vi "Write Top Down Working Set.vi"(8 "error in (no error)":errorcluster, 10 "Top Down Working Set":refnum<data-value>, 11 "Build Analyzer in":refnum<class "Build Analyzer.lvclass">) -> (0 "error out":errorcluster, 3 "Build Analyzer out":refnum<class "Build Analyzer.lvclass">)   [LabVIEW 2017, in "CL_G3_VIComponentBuilder.lvlib" / "Build Analyzer.lvclass"]
doc: "Sets the hierarchy of components in the working set as a LabVIEW Container. Given a node in the tree, the children of this node are returned as dependents."
uses:
  Build Analyzer.lvclass
  <userlib>/_Cirrus Logic/LabVIEW Container/Source/Container/Container.lvclass
  Build Analyzer.lvclass/Build Analyzer.ctl
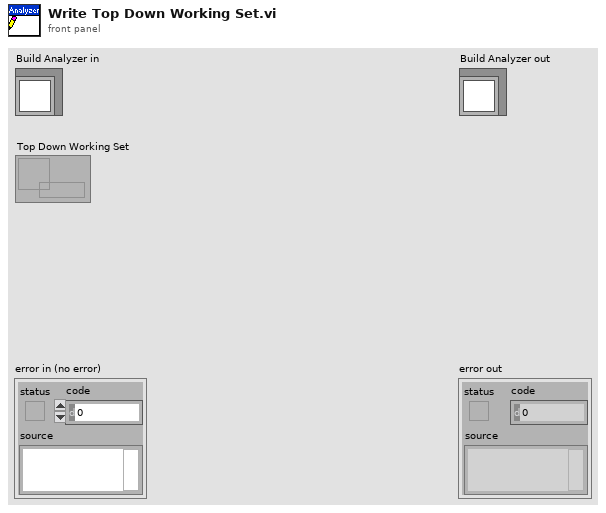
[diagram p1: front panel]
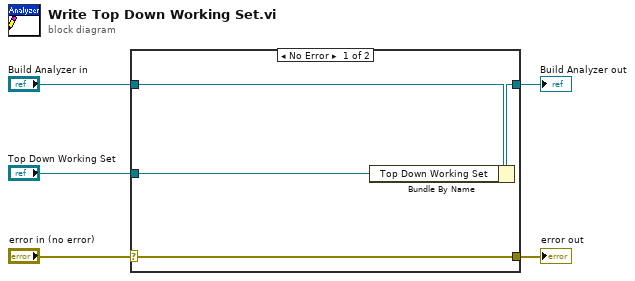
[diagram p0: block diagram]
diagram:
  n1 = case shown="No Error" "error in (no error)" {
    selector: "error in (no error)" -> [w9 w10]
    tunnel: [w9 w10] -> w4
    tunnel: [w7 w11] -> w2
    tunnel: "Build Analyzer in" -> [w8 w11]
    tunnel: "Top Down Working Set" -> [w6 _]
    frame No Error {
      n2 = Bundle By Name(cluster=w8, "Top Down Working Set"=w6) -> (w7:refnum<class "Build Analyzer.lvclass">)
    }
    frame Error {
    }
  }
  "error out" <- w4
  "Build Analyzer out" <- w2
